vi "Flash Align LED.vi"(10 "Thing 2":bool, 11 "Thing 1":bool) -> (3 "Flashy the LED":bool)   [LabVIEW 2011]
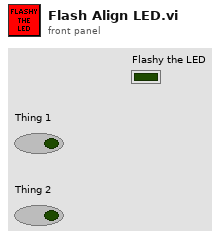
[diagram p1: front panel]
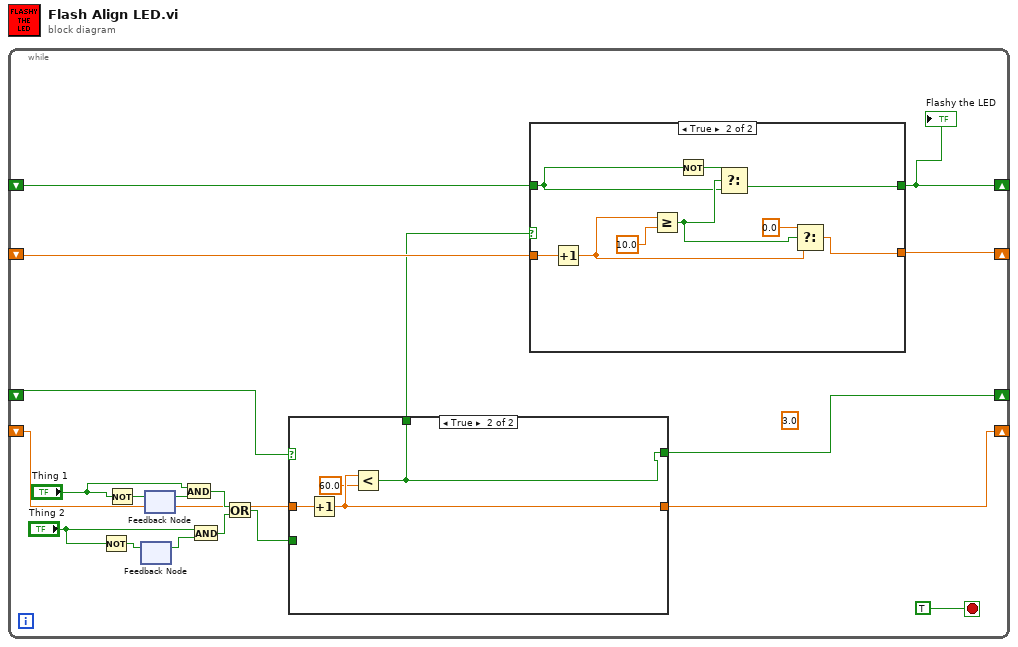
[diagram p0: block diagram]
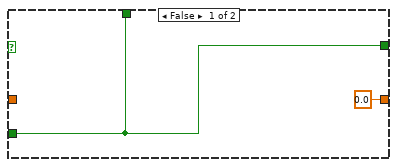
[diagram p2: hidden frame]
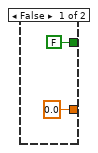
[diagram p3: hidden frame]
diagram:
  (unwired) 3.0 ("y")
  n1 = while {
    shift-right: [w18] -> _
    shift-left: _ -> [w19]
    shift-right: [w8] -> _
    shift-left: _ -> [w7]
    shift-right: [w4] -> _
    shift-left: _ -> [w5]
    shift-right: [w1] -> _
    shift-left: _ -> [w6]
    stop <- TRUE stop-if-true
    n2 = Not(x="Thing 2") -> (.not. x?=w16:bool)
    n3 = Not(x="Thing 1") -> (.not. x?=w17:bool)
    n4 = feedback #1() -> (w15:bool)  [unwired: 1 in]
    n5 = feedback-in #1(w16) -> ()
    n6 = feedback-in #2(w17) -> ()
    n7 = feedback #2() -> (w13:bool)  [unwired: 1 in]
    n8 = And(x="Thing 1", y=w13) -> (x .and. y?=w10:bool)
    n9 = And(x="Thing 2", y=w15) -> (x .and. y?=w11:bool)
    n10 = Or(x=w10, y=w11) -> (x .or. y?=w9:bool)
    n11 = case shown="True" w7 {
      tunnel: [w20 w22] -> w8
      tunnel: w9 -> [w20 _]
      tunnel: w5 -> [_ w25]
      tunnel: [0.0 w24] -> w4
      tunnel: [w20 w22] -> w3
      frame False {
      }
      frame True {
        n12 = Increment(x=w25) -> (x+1=w24:dbl)
        n13 = Less?(x=w24, y=60.0) -> (x < y?=w22:bool)
      }
    }
    n14 = case shown="True" w3 {
      tunnel: w19 -> [_ w36]
      tunnel: [0.0 ("t") w35] -> w18
      tunnel: [FALSE ("Latched") w28] -> w1
      tunnel: w6 -> [_ w29]
      frame False {
      }
      frame True {
        n15 = Increment(x=w36) -> (x+1=w32:dbl)
        n16 = Greater Or Equal?(x=w32, y=10.0) -> (x >= y?=w30:bool)
        n17 = Not(x=w29) -> (.not. x?=w31:bool)
        n18 = Select(t=w31, s=w30, f=w29) -> (s? t:f=w28:bool)
        n19 = Select(t=0.0, s=w30, f=w32) -> (s? t:f=w35:dbl)
      }
    }
    "Flashy the LED" <- w1
  }
